vi "Set Z ROI.vi"(8 "error in (no error)":errorcluster, 11 "Intensity Graph in":refnum<class "TG Graph.lvclass">) -> (0 "error out":errorcluster, 3 "Intensity Graph out":refnum<class "TG Graph.lvclass">)   [LabVIEW 2023]
uses:
  TG Graph/TG Graph.lvclass
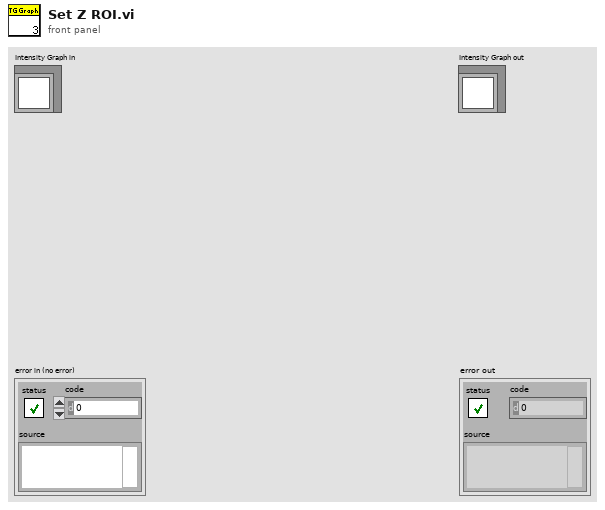
[diagram p1: front panel]
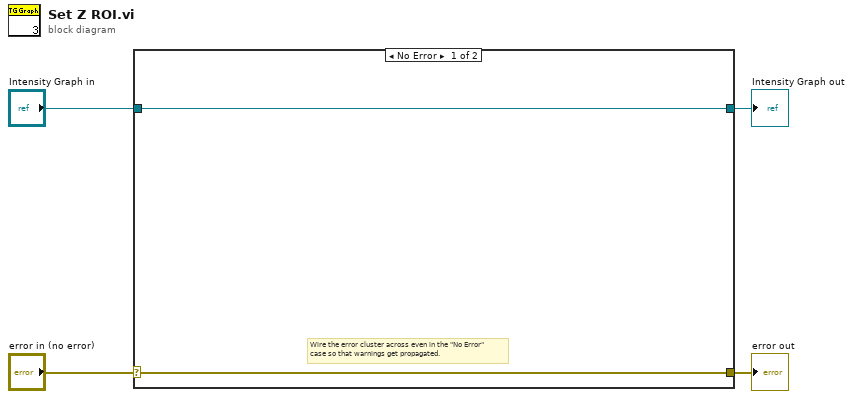
[diagram p0: block diagram]
diagram:
  n1 = case shown="No Error" "error in (no error)" {
    selector: "error in (no error)" -> [w5 w8]
    tunnel: [w5 w8] -> w3
    tunnel: [w6 w7] -> w1
    tunnel: "Intensity Graph in" -> [w6 w7]
    frame No Error {
      # "Wire the error cluster across even in the \"No Error\"\ncase so that warnings get propagated."
    }
    frame Error {
    }
  }
  "error out" <- w3
  "Intensity Graph out" <- w1
